vi "Chrg_Dschrg_1.vi"(0 "Error log filepath":path, 3 "Strain Offset":dbl, 4 "PS VISA in":refnum<visa-resource-name>, 5 "PS error in":errorcluster caption="PS error in (no error)", 6 "CyclePath":path=path "C:/Users/ga11/Desktop/VI/results/3PtestCharge.lvm" caption="Filename", 7 "Battery Type":T1(ring), 8 "Charge/discharge":enum8{"Charge", "Discharge"}(ring), 9 "Charge/Discharge Voltage Setpoint":dbl format="%#.6g", 11 "Current Setpoint":dbl format="%#.6g", 13 "Current Cutoff":dbl) -> (14 "PS VISA out":refnum<visa-resource-name>, 19 "PS error out":errorcluster)   [LabVIEW 2020]
uses:
  <vilib>/Utility/TradDaqScaling.llb/Convert Strain Gauge Reading (scaler).vi
  Drivers-IT-M3400/IT-M3400.lvlib
panel:
  in  "PS error in 2":errorcluster caption="PS error in (no error)"
  out "Read Current(A)":dbl format="%.2g"
  out "Read Voltage(V)":dbl format="%.2g"
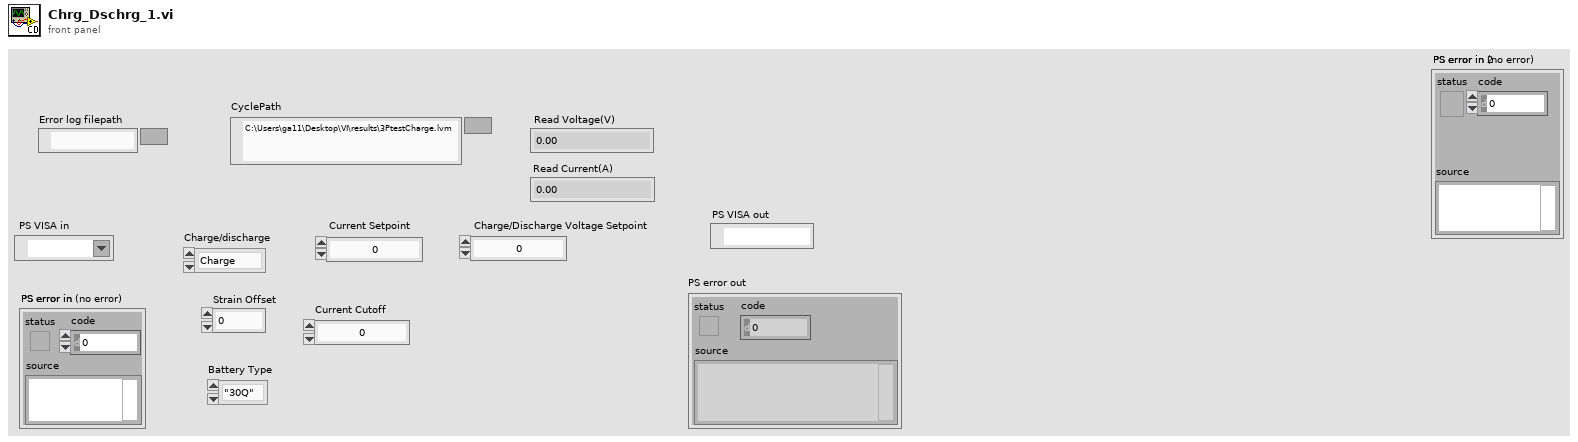
[diagram p1: front panel]
types:
  T1 = enum16{"\"30Q\"", "\"40T\"", "\"2P30Q\"", "\"3P30Q\"", "\"Nissan Leaf\""}
  T2 = cluster{"Baud Rate":u32, "Parity":u16, "Data Bits":u16, "Stop Bits":u16, "Flow Control":u16}
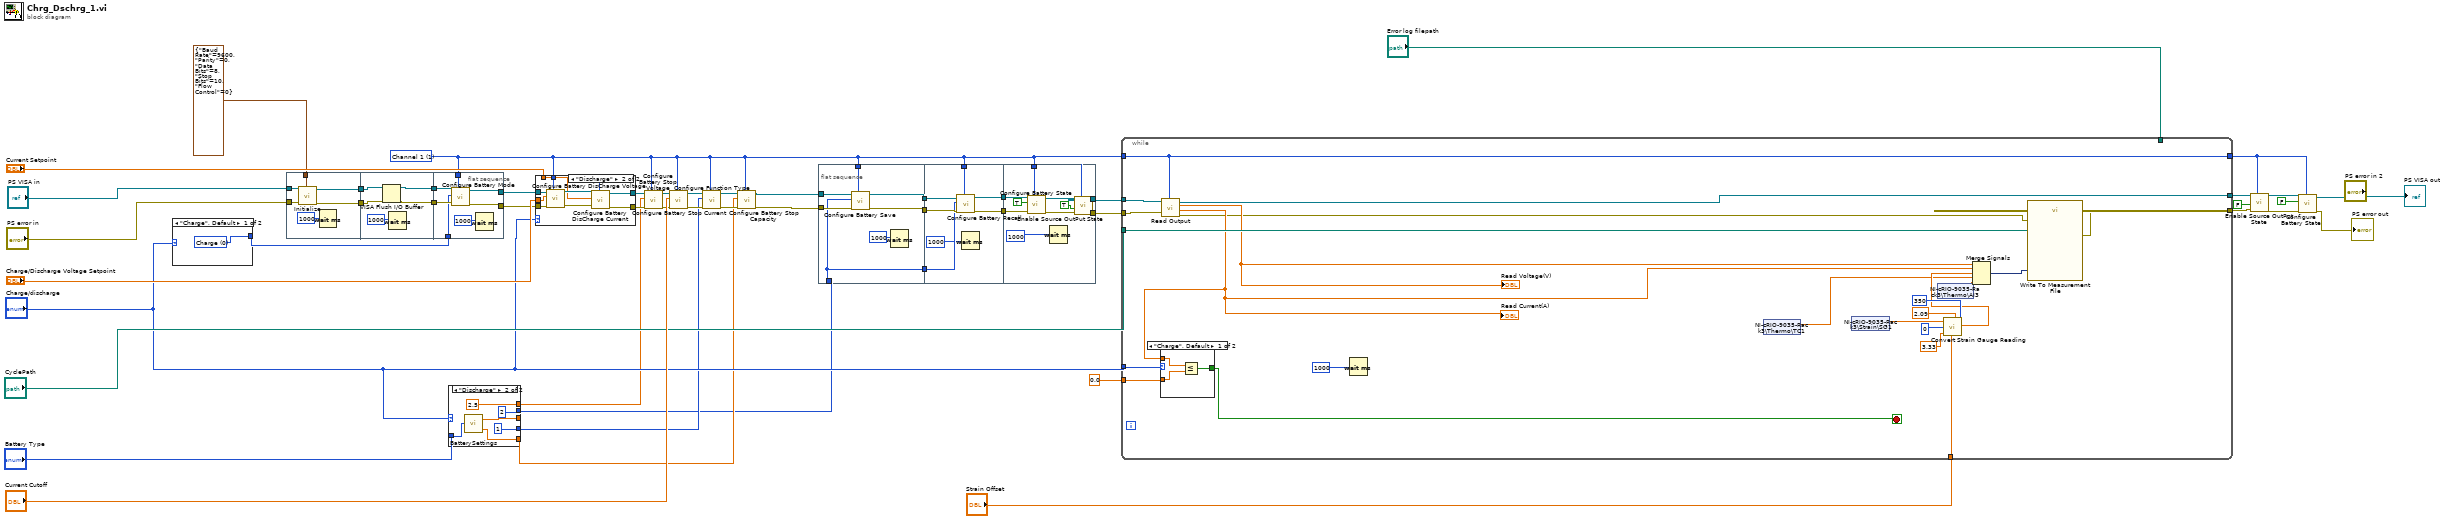
[diagram p0: block diagram]
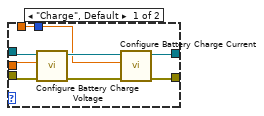
[diagram p2: hidden frame]
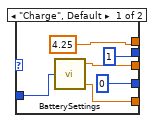
[diagram p3: hidden frame]
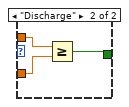
[diagram p4: hidden frame]
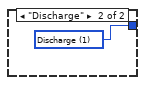
[diagram p5: hidden frame]
diagram:
  w11 = 1 items=["Channel 1"=1, "Channel 2"=2, "Channel 3"=3, "Channel 4"=4, "Channel 5"=5, "Channel 6"=6, "Channel 7"=7, "Channel 8"=8, "Channel 8"=9, "Channel 10"=10, "Channel 11"=11, "Channel 12"=12, "Channel 13"=13, "Channel 14"=14, "Channel 15"=15, "Channel 16"=16] ("Channel")
  n1 = case shown="\"Charge\", Default" "Charge/discharge" {
    tunnel: [w51 w52] -> w19
    frame "Charge", Default {
      w51 = u8 0 items=["Charge", "Discharge"] ("Battery Mode")
    }
    frame "Discharge" {
      w52 = u8 1 items=["Charge", "Discharge"] ("Battery Mode")
    }
  }
  n2 = flat-sequence {
    tunnel: T2 {"Baud Rate"=9600, "Parity"=0, "Data Bits"=8, "Stop Bits"=10, "Flow Control"=0} ("Serial Configuration") -> [w58]
    tunnel: "PS error in" -> [w57]
    tunnel: "PS VISA in" -> [w56]
    tunnel: [w54] -> w5
    tunnel: [w53] -> w4
    tunnel: [w60] -> w35
    tunnel: [w59] -> w34
    tunnel: w5 -> [w62]
    tunnel: w4 -> [w61]
    tunnel: w35 -> [w67]
    tunnel: w34 -> [w69]
    tunnel: w11 -> [w70]
    tunnel: w19 -> [w68]
    tunnel: [w64] -> w8
    tunnel: [w65] -> w7
    frame #0 {
      n3 = call "Initialize.vi"("Serial Configuration"=w58, "error in"=w57, "VISA resource name"=w56) -> ("error out"=w53:errorcluster, "VISA resource name out"=w54:refnum<visa-resource-name>)  [unwired: 7 in]
      n4 = Wait (ms)(milliseconds to wait=1000) -> ()  [unwired: 1 out]
    }
    frame #1 {
      n5 = VISA Flush I/O Buffer(VISA resource name=w62, error in (no error)=w61) -> (VISA resource name out=w60:refnum<visa-resource-name>, error out=w59:errorcluster)  [unwired: 1 in]
      n6 = Wait (ms)(milliseconds to wait=1000) -> ()  [unwired: 1 out]
    }
    frame #2 {
      n7 = call "Configure Battery Mode.vi"("Channel"=w70, "error in"=w69, "Battery Mode"=w68, "VISA resource name"=w67) -> ("error out"=w64:errorcluster, "VISA resource name out"=w65:refnum<visa-resource-name>)  [unwired: 6 in]
      n8 = Wait (ms)(milliseconds to wait=1000) -> ()  [unwired: 1 out]
    }
  }
  n9 = case shown="\"Discharge\"" "Charge/discharge" {
    tunnel: "Battery Type" -> [w76 w82]
    tunnel: [w75 w80] -> _
    tunnel: [u8 0 ("File") u8 1 ("File")] -> w13
    tunnel: [u8 1 ("File") u8 2 ("File")] -> w10
    tunnel: [w72 w78] -> w12
    tunnel: [4.25 2.5] -> w9
    frame "Charge", Default {
      n10 = call "BatterySettings.vi"("Battery Type"=w76) -> ("RatedCapacity (Ah)"=w72:dbl, "Max Voltage (V)"=w75:dbl)  [unwired: 2 in, 1 out]
    }
    frame "Discharge" {
      n11 = call "BatterySettings.vi"("Battery Type"=w82) -> ("RatedCapacity (Ah)"=w78:dbl, "Min Voltage (V)"=w80:dbl)  [unwired: 2 in, 1 out]
    }
  }
  n12 = case shown="\"Discharge\"" "Charge/discharge" {
    tunnel: w7 -> [w90 w99]
    tunnel: w8 -> [w89 w98]
    tunnel: [w84 w95] -> w27
    tunnel: [w83 w94] -> w26
    tunnel: w11 -> [_ w93]
    tunnel: "Charge/Discharge Voltage Setpoint" -> [w86 w92]
    tunnel: "Current Setpoint" -> [w85 w91]
    frame "Charge", Default {
      n13 = call "Configure Battery Charge Voltage.vi"("error in"=w89, "Charge Voltage(V)"=w86, "VISA resource name"=w90) -> ("error out"=w87:errorcluster, "VISA resource name out"=w88:refnum<visa-resource-name>)  [unwired: 6 in]
      n14 = call "Configure Battery Charge Current.vi"("error in"=w87, "Charge Current(A)"=w85, "VISA resource name"=w88) -> ("error out"=w83:errorcluster, "VISA resource name out"=w84:refnum<visa-resource-name>)  [unwired: 7 in]
    }
    frame "Discharge" {
      n15 = call "Configure Battery DisCharge Voltage.vi"("Channel"=w93, "error in"=w98, "Discharge Voltage(V)"=w92, "VISA resource name"=w99) -> ("error out"=w96:errorcluster, "VISA resource name out"=w97:refnum<visa-resource-name>)  [unwired: 6 in]
      n16 = call "Configure Battery DisCharge Current.vi"("Channel"=w93, "error in"=w96, "Discharge Current(A)"=w91, "VISA resource name"=w97) -> ("error out"=w94:errorcluster, "VISA resource name out"=w95:refnum<visa-resource-name>)  [unwired: 6 in]
    }
  }
  n17 = call "Configure Battery Stop Voltage.vi"("Channel"=w11, "error in"=w26, "Stop Voltage(V)"=w9, "VISA resource name"=w27) -> ("error out"=w32:errorcluster, "VISA resource name out"=w33:refnum<visa-resource-name>)  [unwired: 6 in]
  n18 = call "Configure Battery Stop Current.vi"("Channel"=w11, "error in"=w32, "Stop Current(A)"="Current Cutoff", "VISA resource name"=w33) -> ("error out"=w15:errorcluster, "VISA resource name out"=w17:refnum<visa-resource-name>)  [unwired: 6 in]
  n19 = call "Configure Function Type.vi"("Channel"=w11, "error in"=w15, "Function Type"=w13, "VISA resource name"=w17) -> ("error out"=w14:errorcluster, "VISA resource name out"=w16:refnum<visa-resource-name>)  [unwired: 6 in]
  n20 = call "Configure Battery Stop Capacity.vi"("Channel"=w11, "error in"=w14, "Stop Capacity(Ah)"=w12, "VISA resource name"=w16) -> ("error out"=w2:errorcluster, "VISA resource name out"=w3:refnum<visa-resource-name>)  [unwired: 6 in]
  n21 = flat-sequence {
    tunnel: w10 -> [w105]
    tunnel: w11 -> [w100]
    tunnel: [w103] -> w40
    tunnel: [w105] -> w39
    tunnel: [w102] -> w38
    tunnel: w2 -> [w106]
    tunnel: w3 -> [w104]
    tunnel: [w109] -> w37
    tunnel: [w110] -> w36
    tunnel: w40 -> [w113]
    tunnel: w39 -> [w112]
    tunnel: w38 -> [w111]
    tunnel: w11 -> [w107]
    tunnel: [w117] -> w25
    tunnel: [w116] -> w24
    tunnel: w11 -> [w115]
    tunnel: w37 -> [w123]
    tunnel: w36 -> [w122]
    frame #0 {
      n22 = call "Configure Battery Save.vi"("Channel"=w100, "error in"=w106, "File"=w105, "VISA resource name"=w104) -> ("error out"=w103:errorcluster, "VISA resource name out"=w102:refnum<visa-resource-name>)  [unwired: 6 in]
      n23 = Wait (ms)(milliseconds to wait=1000) -> ()  [unwired: 1 out]
    }
    frame #1 {
      n24 = call "Configure Battery Recall.vi"("Channel"=w107, "error in"=w113, "File"=w112, "VISA resource name"=w111) -> ("error out"=w110:errorcluster, "VISA resource name out"=w109:refnum<visa-resource-name>)  [unwired: 6 in]
      n25 = Wait (ms)(milliseconds to wait=1000) -> ()  [unwired: 1 out]
    }
    frame #2 {
      n26 = call "Configure Battery State.vi"("Channel"=w115, "error in"=w122, "State"=TRUE, "VISA resource name"=w123) -> ("error out"=w120:errorcluster, "VISA resource name out"=w121:refnum<visa-resource-name>)  [unwired: 6 in]
      n27 = Wait (ms)(milliseconds to wait=1000) -> ()  [unwired: 1 out]
      n28 = call "Enable Source OutPut State.vi"("Channel"=w115, "error in"=w120, "State"=TRUE ("Enable Output|Intput"), "VISA resource name"=w121) -> ("error out"=w116:errorcluster, "VISA resource name out"=w117:refnum<visa-resource-name>)  [unwired: 6 in]
    }
  }
  n29 = while {
    tunnel: [w139] -> w23
    tunnel: [w127] -> w22
    tunnel: w25 -> [w146]
    tunnel: w24 -> [w145]
    tunnel: w11 -> [w129]
    tunnel: [w129] -> w21
    tunnel: "CyclePath" -> [w143]
    tunnel: 0.0 -> [w141]
    tunnel: "Charge/discharge" -> [w140]
    tunnel: "Strain Offset" -> [w134]
    tunnel: "Error log filepath" -> [_]
    stop <- w133 stop-if-true
    n30 = call "Read Output.vi"("Channel"=w129, "error in"=w145, "VISA resource name"=w146) -> ("error out"=w128:errorcluster, "Read Current(A)"=w130:dbl, "Read Voltage(V)"=w131:dbl, "VISA resource name out"=w139:refnum<visa-resource-name>)  [unwired: 5 in]
    "Read Voltage(V)" <- w131
    "Read Current(A)" <- w130
    n31 = case shown="\"Charge\", Default" w140 {
      tunnel: w141 -> [w148 w151]
      tunnel: w130 -> [w149 w152]
      tunnel: [w147 w150] -> w133
      frame "Charge", Default {
        n32 = Less Or Equal?(x=w149, y=w148) -> (x <= y?=w147:bool)
      }
      frame "Discharge" {
        n33 = Greater Or Equal?(x=w152, y=w151) -> (x >= y?=w150:bool)
      }
    }
    n34 = Wait (ms)(milliseconds to wait=1000) -> ()  [unwired: 1 out]
    n35 = shared-variable "NI-cRIO-9035-Rack3\\Thermo\\TC1"() -> (w124:dbl)  [unwired: 1 in, 1 out]
    n36 = shared-variable "NI-cRIO-9035-Rack3\\Strain\\SG1"() -> (w132:dbl)  [unwired: 1 in, 1 out]
    n37 = shared-variable "NI-cRIO-9035-Rack3\\Thermo\\AI3"() -> (w125:dbl)  [unwired: 1 in, 1 out]
    n38 = call-poly <vilib>:"Convert Strain Gauge Reading.vi"("Vsg (0.0)"=w132, "Bridge Configuration\n(3:Half Bridge II)"=0, "Vex (3.33)"=3.33, "Vinit (0.0)"=w134, "GF (2.0)"=2.09, "Rg (120)"=350) -> ("Strain"=w126:sgl)  [unwired: 4 in]
    n39 = Merge Signals "Merge Signals"(w131, w130, w126, w124, w125) -> (w144:dynamicdata)
    n40 = call "Write To Measurement File"("Signals"=w144, "error in (no error)"=w128, "Filename"=w143) -> ("error out"=w127:errorcluster)  [unwired: 14 in, 2 out]
  }
  n41 = call "Enable Source OutPut State.vi"("Channel"=w21, "error in"=w22, "State"=FALSE, "VISA resource name"=w23) -> ("error out"=w30:errorcluster, "VISA resource name out"=w31:refnum<visa-resource-name>)  [unwired: 6 in]
  n42 = call "Configure Battery State.vi"("Channel"=w21, "error in"=w30, "State"=FALSE, "VISA resource name"=w31) -> ("error out"=→"PS error out":errorcluster, "VISA resource name out"=→"PS VISA out":refnum<visa-resource-name>)  [unwired: 6 in]
